vi "Read Step State.vi"(8 "error in (no error)":errorcluster, 11 "Result in":refnum<class "Result.lvclass">) -> (0 "error out":errorcluster, 2 "Step State":T1, 3 "Result out":refnum<class "Result.lvclass">)   [LabVIEW 2015, in "Result.lvclass"]
uses:
  Result.lvclass
  Step/Execution/Step Status.ctl
  Result.lvclass/Result.ctl
  Step/Execution/Step.lvclass
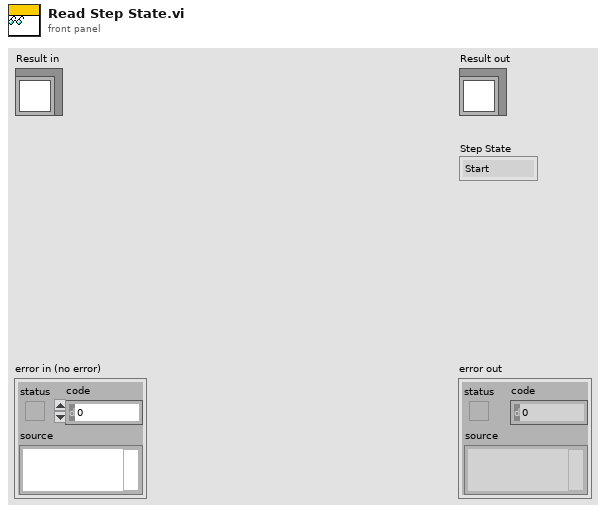
[diagram p1: front panel]
types:
  T1 = typedef "Step.lvclass/Step Status.ctl" = enum16{"Start", "Passed", "Failed", "Error", "Done", "Terminated", "Skipped", "Running"}
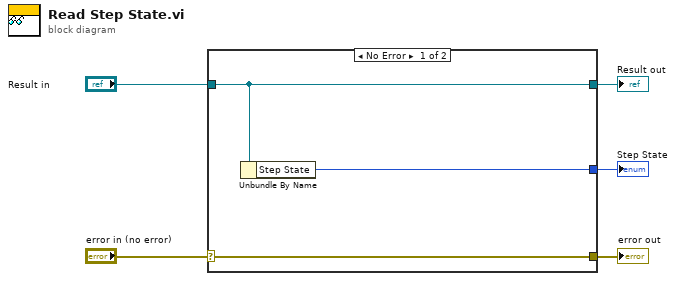
[diagram p0: block diagram]
diagram:
  n1 = case shown="No Error" "error in (no error)" {
    selector: "error in (no error)" -> [w8 w9]
    tunnel: [w8 w9] -> w4
    tunnel: [w7 w10] -> w2
    tunnel: "Result in" -> [w7 w10]
    tunnel: [w6 _] -> w1
    frame No Error {
      n2 = Unbundle By Name(w7) -> ("Step State"=w6:T1)
    }
    frame Error {
    }
  }
  "error out" <- w4
  "Result out" <- w2
  "Step State" <- w1
